vi "Process Build VI Operation.vi"(6 "Caller VI Path":path, 7 "Assert Scripting Configuration":T1, 8 "error in (no error)":errorcluster, 10 "Discard?":bool) -> (0 "error out":errorcluster, 3 "Assert VI Path":path, 5 "Valid Configuration":bool)   [LabVIEW 2016]
uses:
  Assert Scripting Configuration.ctl
  <vilib>/Utility/Data Type/Type Definitions/Data Type.ctl
  <vilib>/Utility/Data Type/NI_Data Type.lvlib
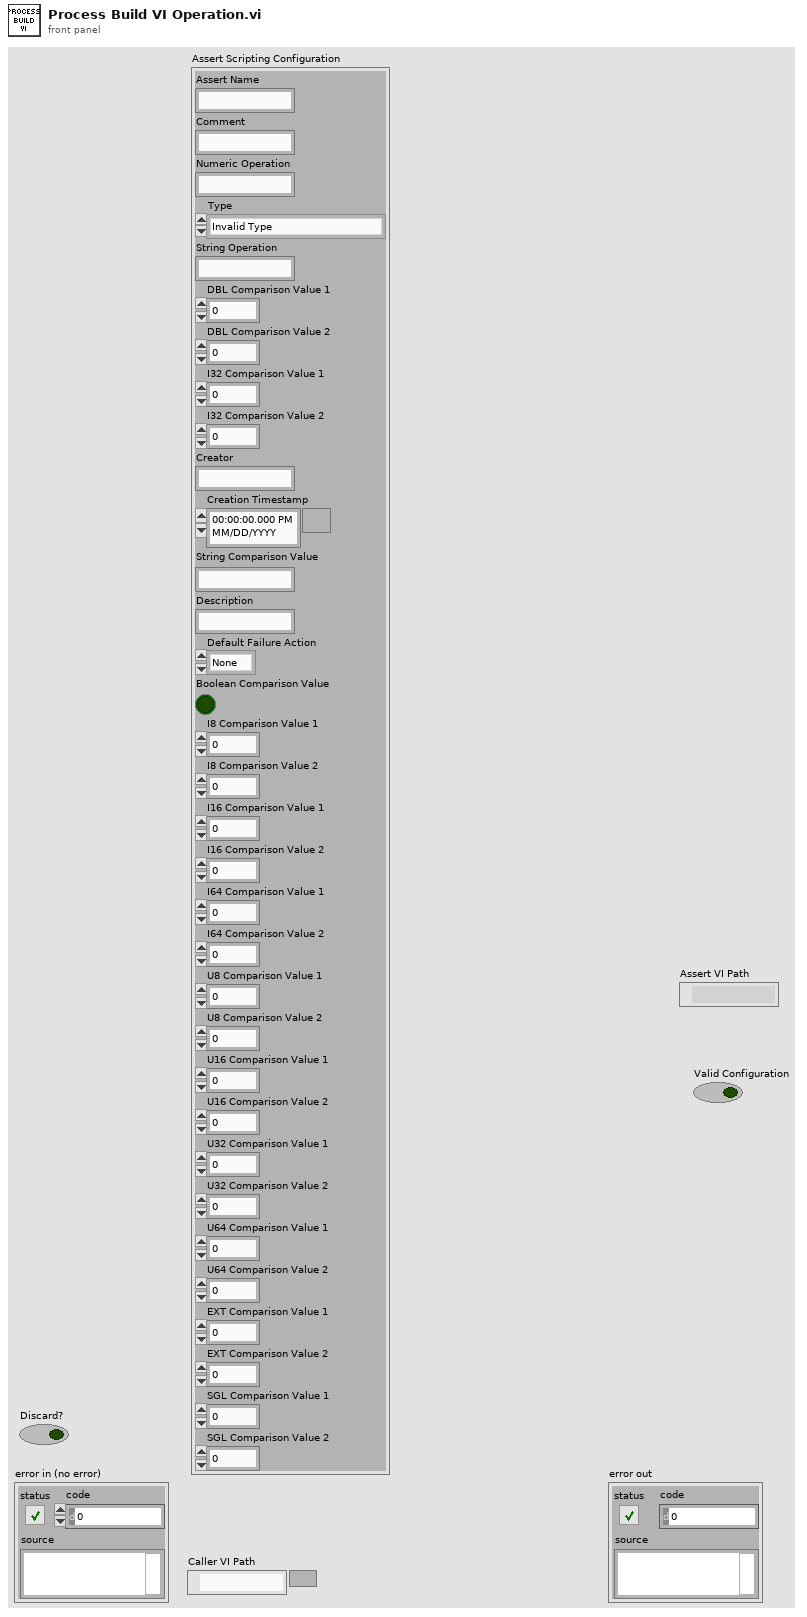
[diagram p1: front panel]
types:
  T1 = typedef "Assert Scripting Configuration.ctl" = cluster{"Assert Name":string, "Comment":string, "Numeric Operation":string, "Type":T2, "String Operation":string, "DBL Comparison Value 1":dbl, "DBL Comparison Value 2":dbl, "I32 Comparison Value 1":i32, "I32 Comparison Value 2":i32, "Creator":string, "Creation Timestamp":timestamp, "String Comparison Value":string, "Description":string, "Default Failure Action":enum16{"None", "Log To File", "Pause Execution", "Abort Execution"}, "Boolean Comparison Value":bool, "I8 Comparison Value 1":i8, "I8 Comparison Value 2":i8, "I16 Comparison Value 1":i16, "I16 Comparison Value 2":i16, "I64 Comparison Value 1":i64, "I64 Comparison Value 2":i64, "U8 Comparison Value 1":u8, "U8 Comparison Value 2":u8, "U16 Comparison Value 1":u16, "U16 Comparison Value 2":u16, "U32 Comparison Value 1":u32, "U32 Comparison Value 2":u32, "U64 Comparison Value 1":u64, "U64 Comparison Value 2":u64, "EXT Comparison Value 1":ext, "EXT Comparison Value 2":ext, "SGL Comparison Value 1":sgl, "SGL Comparison Value 2":sgl}
  T2 = typedef "NI_Data Type.lvlib/Data Type.ctl" = enum8{"Invalid Type", "Void", "I8", "I16", "I32", "I64", "U8", "U16", "U32", "U64", "Single Float", "Double Float", "Extended Float", "Single Complex", "Double Complex", "Extended Complex", "Enum U8", "Enum U16", "Enum U32", "Enum U64", "Single Float With Unit", "Double Float With Unit", "Extended Float With Unit", "Single Complex with Unit", "Double Complex with Unit", "Extended Complex with Unit", "Boolean", "String", "Path", "Picture", "Tag", "Array", "Cluster", "Variant", "LV Variant", "Waveform", "Timestamp", "Digital Waveform", "Digital Data", "ExpressData", "Refnum", "External Data", "VI", "Poly VI", "LabVIEW Class Instance", "Fixed Point"}
  T3 = enum16{"None", "Log To File", "Pause Execution", "Abort Execution"}
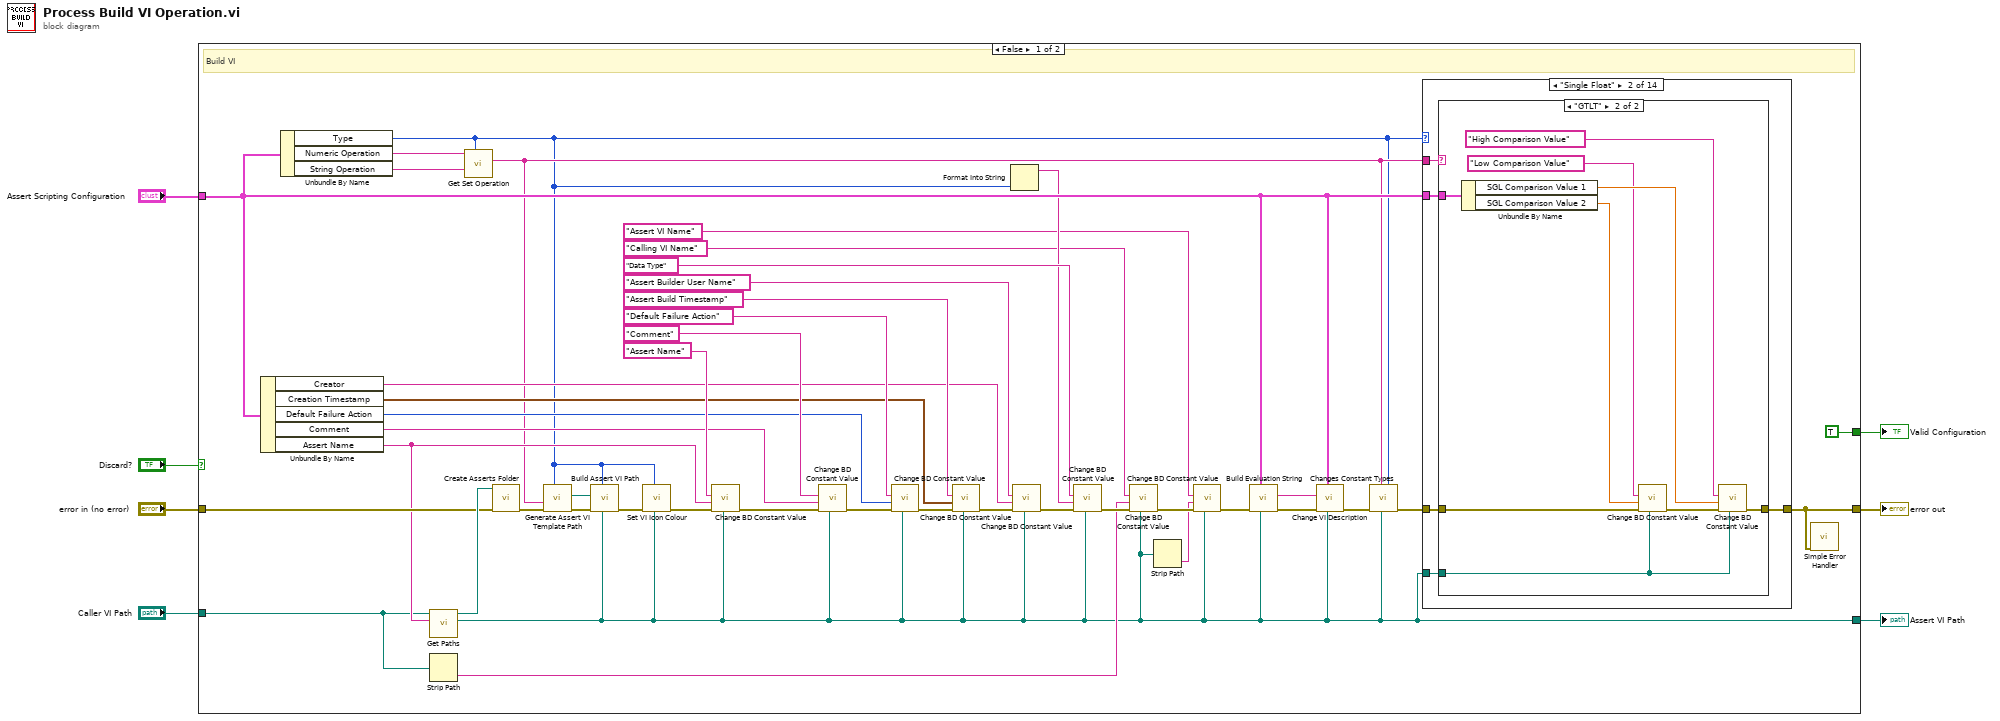
[diagram p0: block diagram]
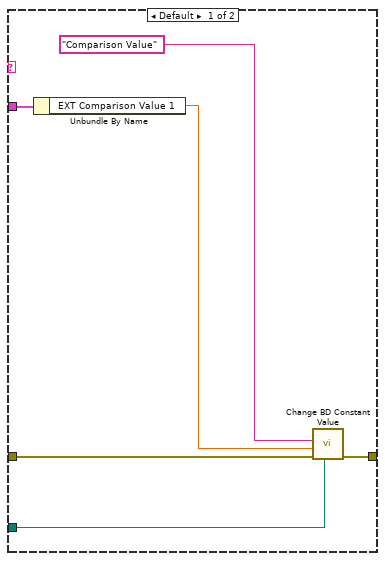
[diagram p3: hidden frame]
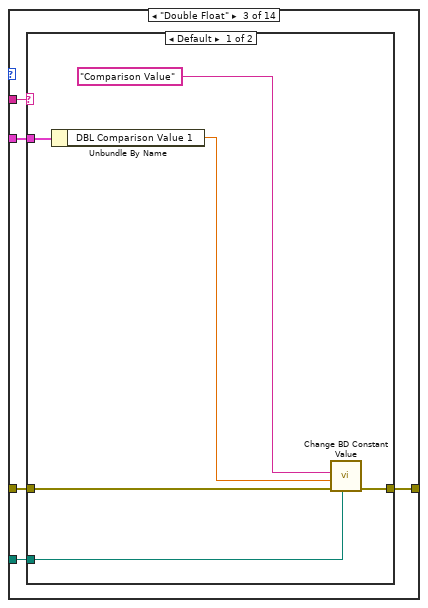
[diagram p4: hidden frame]
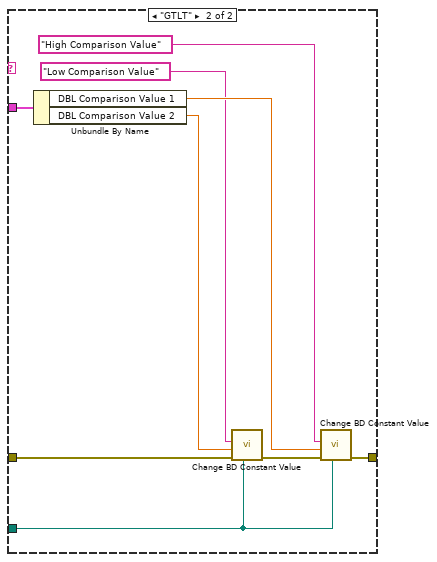
[diagram p5: hidden frame]
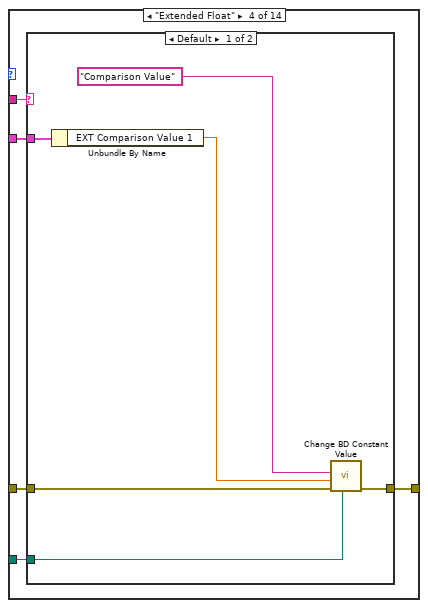
[diagram p6: hidden frame]
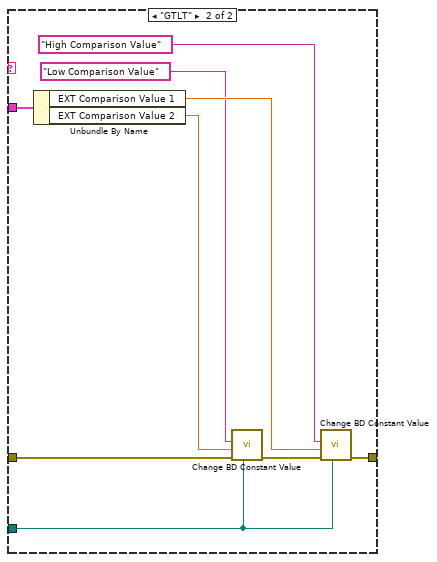
[diagram p7: hidden frame]
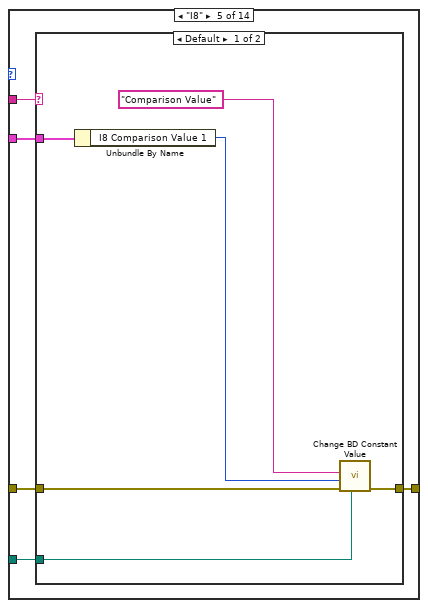
[diagram p8: hidden frame]
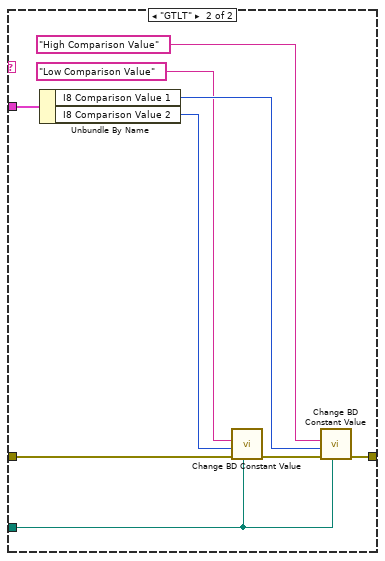
[diagram p9: hidden frame]
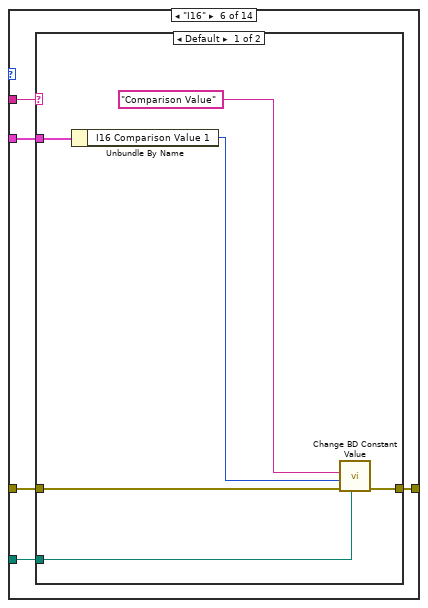
[diagram p10: hidden frame]
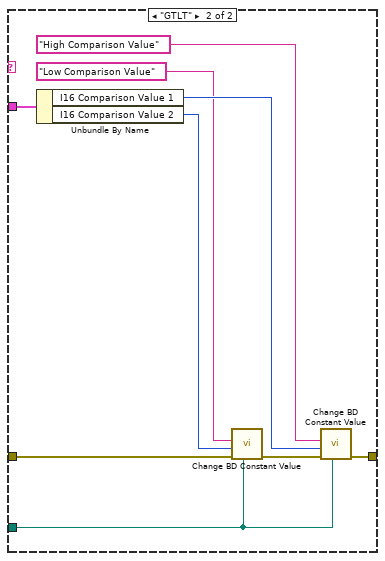
[diagram p11: hidden frame]
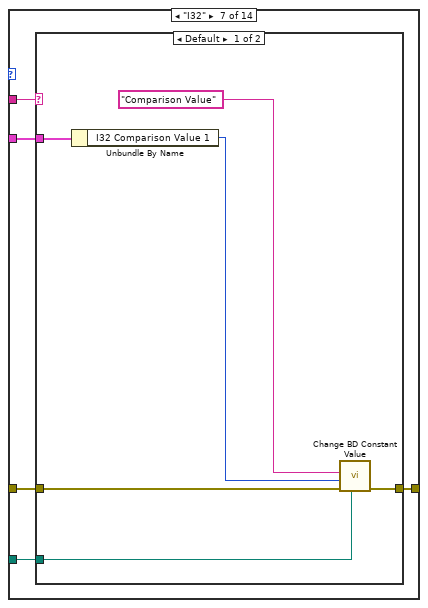
[diagram p12: hidden frame]
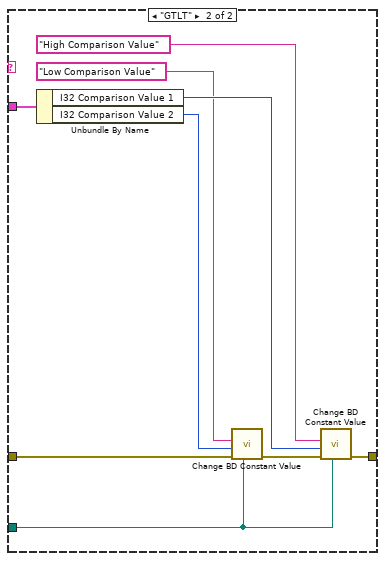
[diagram p13: hidden frame]
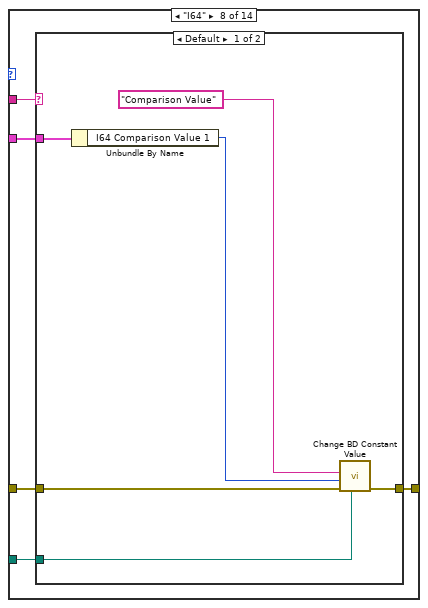
[diagram p14: hidden frame]
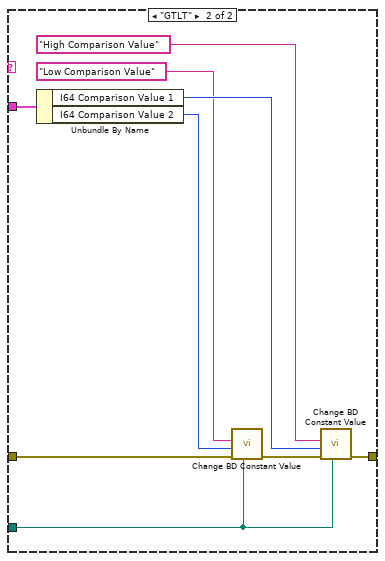
[diagram p15: hidden frame]
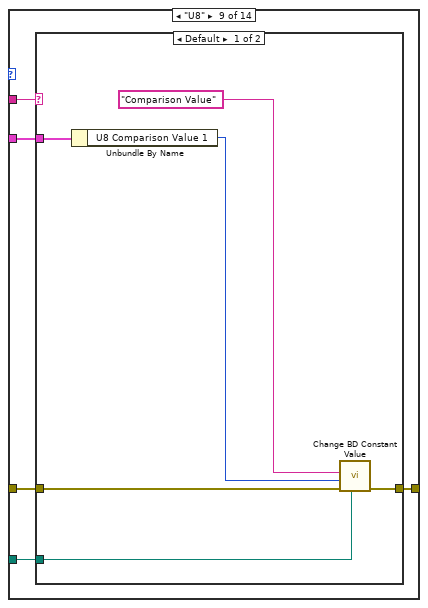
[diagram p16: hidden frame]
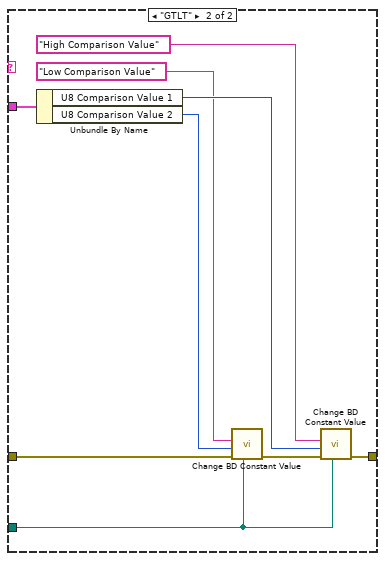
[diagram p17: hidden frame]
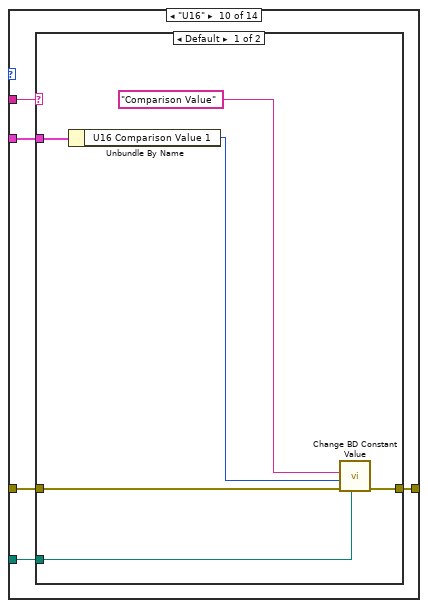
[diagram p18: hidden frame]
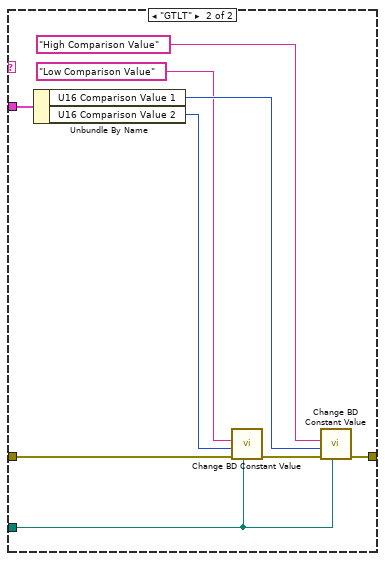
[diagram p19: hidden frame]
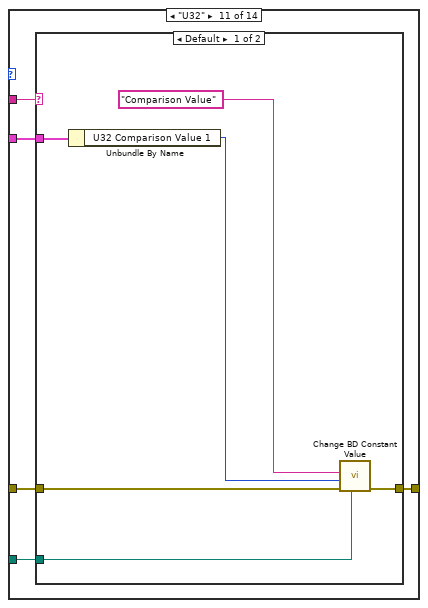
[diagram p20: hidden frame]
diagram:
  n1 = case shown="False" "Discard?" {
    tunnel: "error in (no error)" -> [w43 w285]
    tunnel: "Caller VI Path" -> [w15 _]
    tunnel: [w30 w285] -> w4
    tunnel: [w9 _] -> w5
    tunnel: [TRUE _] -> w6
    tunnel: "Assert Scripting Configuration" -> [w32 _]
    frame False {
      # "Build VI"
      n2 = Unbundle By Name(w32) -> ("Creator"=w21:string, "Creation Timestamp"=w22:timestamp, "Default Failure Action"=w34:T3, "Comment"=w37:string, "Assert Name"=w38:string)
      n3 = Unbundle By Name(w32) -> ("Type"=w8:T2, "Numeric Operation"=w40:string, "String Operation"=w39:string)
      n4 = call "Get Paths.vi"("Assert Name"=w38, "Path"=w15) -> ("Assert VI Path"=w9:path, "Asserts Folder Path"=w50:path)  [unwired: 8 in]
      n5 = Strip Path(path=w15) -> (name=w14:string)  [unwired: 1 out]
      n6 = call "Get Set Operation.vi"("Type"=w8, "String Operation"=w39, "Numeric Operation"=w40) -> ("Operation"=w10:string)  [unwired: 8 in]
      n7 = call "Create Asserts Folder.vi"("error in (no error)"=w43, "Folder Path"=w50) -> ("error out"=w44:errorcluster)  [unwired: 9 in]
      n8 = call "Generate Assert VI Template Path.vi"("Data Type"=w8, "error in (no error)"=w44, "Operation"=w10) -> ("error out"=w42:errorcluster, "Template Path"=w41:path)  [unwired: 7 in]
      n9 = call "Build Assert VI Path.vi"("Assert VI path"=w9, "Type"=w8, "error in (no error)"=w42, "Template Path"=w41) -> ("error out"=w51:errorcluster)  [unwired: 7 in]
      n10 = call "Set VI Icon Colour.vi"("VI Path"=w9, "Type"=w8, "error in (no error)"=w51) -> ("error out"=w13:errorcluster)  [unwired: 8 in]
      n11 = call "Change BD Constant Value.vi"("Assert VI Path"=w9, "error in (no error)"=w13, "Data Value"=w38, "Constant Name"="Assert Name") -> ("error out"=w46:errorcluster)  [unwired: 7 in]
      n12 = call "Change BD Constant Value.vi"("Assert VI Path"=w9, "error in (no error)"=w46, "Data Value"=w37, "Constant Name"="Comment") -> ("error out"=w45:errorcluster)  [unwired: 7 in]
      n13 = call "Change BD Constant Value.vi"("Assert VI Path"=w9, "error in (no error)"=w45, "Data Value"=w34, "Constant Name"="Default Failure Action") -> ("error out"=w36:errorcluster)  [unwired: 7 in]
      n14 = call "Change BD Constant Value.vi"("Assert VI Path"=w9, "error in (no error)"=w36, "Data Value"=w22, "Constant Name"="Assert Build Timestamp") -> ("error out"=w28:errorcluster)  [unwired: 7 in]
      n15 = Format Into String(w8) -> (resulting string=w23:string)  [unwired: 3 in, 1 out]
      n16 = call "Change BD Constant Value.vi"("Assert VI Path"=w9, "error in (no error)"=w28, "Data Value"=w21, "Constant Name"="Assert Builder User Name") -> ("error out"=w29:errorcluster)  [unwired: 7 in]
      n17 = call "Change BD Constant Value.vi"("Assert VI Path"=w9, "error in (no error)"=w29, "Data Value"=w23, "Constant Name"="Data Type") -> ("error out"=w27:errorcluster)  [unwired: 7 in]
      n18 = call "Change BD Constant Value.vi"("Assert VI Path"=w9, "error in (no error)"=w27, "Data Value"=w14, "Constant Name"="Calling VI Name") -> ("error out"=w20:errorcluster)  [unwired: 7 in]
      n19 = Strip Path(path=w9) -> (name=w16:string)  [unwired: 1 out]
      n20 = call "Change BD Constant Value.vi"("Assert VI Path"=w9, "error in (no error)"=w20, "Data Value"=w16, "Constant Name"="Assert VI Name") -> ("error out"=w19:errorcluster)  [unwired: 7 in]
      n21 = call "Build Evaluation String.vi"("VI Path"=w9, "Assert Scripting Configuration"=w32, "error in (no error)"=w19) -> ("error out"=w33:errorcluster, "Evaluation String"=w31:string)  [unwired: 7 in]
      n22 = call "Change VI Description.vi"("VI Path"=w9, "Assert Scripting Configuration"=w32, "error in (no error)"=w33, "Evaluation String"=w31) -> ("error out"=w12:errorcluster)  [unwired: 7 in]
      n23 = call "Changes Constant Types.vi"("Requested Data Type"=w8, "Assert VI Path"=w9, "String Control Name"=w10, "error in (no error)"=w12) -> ("error out"=w11:errorcluster)  [unwired: 7 in]
      n24 = case shown="\"Single Float\"" w8 {
        tunnel: w9 -> [_ w55 w75 w95 w117 w137 w157 w177 w197 w217 w237 w257 w274 w280]
        tunnel: w11 -> [w52 w56 w76 w96 w116 w136 w156 w176 w196 w216 w236 w256 w278 w284]
        tunnel: [w52 w57 w77 w97 w115 w135 w155 w175 w195 w215 w235 w255 w277 w283] -> w30
        tunnel: w32 -> [_ w54 w74 w94 w114 w134 w154 w174 w194 w214 w234 w254 w276 w282]
        tunnel: w10 -> [_ w53 w73 w93 w113 w133 w153 w173 w193 w213 w233 w253 _ _]
        frame Default {
        }
        frame "Single Float" {
          n25 = case shown="\"GTLT\"" w53 {
            tunnel: w55 -> [w58 w64]
            tunnel: w56 -> [w63 w72]
            tunnel: [w62 w68] -> w57
            tunnel: w54 -> [w61 w70]
            frame Default {
              n26 = Unbundle By Name(w61) -> ("EXT Comparison Value 1"=w60:ext)
              n27 = call "Change BD Constant Value.vi"("Assert VI Path"=w58, "error in (no error)"=w63, "Data Value"=w60, "Constant Name"="Comparison Value") -> ("error out"=w62:errorcluster)  [unwired: 7 in]
            }
            frame "GTLT" {
              n28 = Unbundle By Name(w70) -> ("SGL Comparison Value 1"=w67:sgl, "SGL Comparison Value 2"=w69:sgl)
              n29 = call "Change BD Constant Value.vi"("Assert VI Path"=w64, "error in (no error)"=w72, "Data Value"=w69, "Constant Name"="Low Comparison Value") -> ("error out"=w71:errorcluster)  [unwired: 7 in]
              n30 = call "Change BD Constant Value.vi"("Assert VI Path"=w64, "error in (no error)"=w71, "Data Value"=w67, "Constant Name"="High Comparison Value") -> ("error out"=w68:errorcluster)  [unwired: 7 in]
            }
          }
        }
        frame "Double Float" {
          n31 = case shown="Default" w73 {
            tunnel: w75 -> [w78 w84]
            tunnel: w76 -> [w83 w92]
            tunnel: [w82 w88] -> w77
            tunnel: w74 -> [w81 w90]
            frame Default {
              n32 = Unbundle By Name(w81) -> ("DBL Comparison Value 1"=w80:dbl)
              n33 = call "Change BD Constant Value.vi"("Assert VI Path"=w78, "error in (no error)"=w83, "Data Value"=w80, "Constant Name"="Comparison Value") -> ("error out"=w82:errorcluster)  [unwired: 7 in]
            }
            frame "GTLT" {
              n34 = Unbundle By Name(w90) -> ("DBL Comparison Value 1"=w87:dbl, "DBL Comparison Value 2"=w89:dbl)
              n35 = call "Change BD Constant Value.vi"("Assert VI Path"=w84, "error in (no error)"=w92, "Data Value"=w89, "Constant Name"="Low Comparison Value") -> ("error out"=w91:errorcluster)  [unwired: 7 in]
              n36 = call "Change BD Constant Value.vi"("Assert VI Path"=w84, "error in (no error)"=w91, "Data Value"=w87, "Constant Name"="High Comparison Value") -> ("error out"=w88:errorcluster)  [unwired: 7 in]
            }
          }
        }
        frame "Extended Float" {
          n37 = case shown="Default" w93 {
            tunnel: w95 -> [w98 w104]
            tunnel: w96 -> [w103 w112]
            tunnel: [w102 w108] -> w97
            tunnel: w94 -> [w101 w110]
            frame Default {
              n38 = Unbundle By Name(w101) -> ("EXT Comparison Value 1"=w100:ext)
              n39 = call "Change BD Constant Value.vi"("Assert VI Path"=w98, "error in (no error)"=w103, "Data Value"=w100, "Constant Name"="Comparison Value") -> ("error out"=w102:errorcluster)  [unwired: 7 in]
            }
            frame "GTLT" {
              n40 = Unbundle By Name(w110) -> ("EXT Comparison Value 1"=w107:ext, "EXT Comparison Value 2"=w109:ext)
              n41 = call "Change BD Constant Value.vi"("Assert VI Path"=w104, "error in (no error)"=w112, "Data Value"=w109, "Constant Name"="Low Comparison Value") -> ("error out"=w111:errorcluster)  [unwired: 7 in]
              n42 = call "Change BD Constant Value.vi"("Assert VI Path"=w104, "error in (no error)"=w111, "Data Value"=w107, "Constant Name"="High Comparison Value") -> ("error out"=w108:errorcluster)  [unwired: 7 in]
            }
          }
        }
        frame "I8" {
          n43 = case shown="Default" w113 {
            tunnel: w117 -> [w118 w124]
            tunnel: w116 -> [w123 w132]
            tunnel: [w122 w128] -> w115
            tunnel: w114 -> [w121 w130]
            frame Default {
              n44 = Unbundle By Name(w121) -> ("I8 Comparison Value 1"=w120:i8)
              n45 = call "Change BD Constant Value.vi"("Assert VI Path"=w118, "error in (no error)"=w123, "Data Value"=w120, "Constant Name"="Comparison Value") -> ("error out"=w122:errorcluster)  [unwired: 7 in]
            }
            frame "GTLT" {
              n46 = Unbundle By Name(w130) -> ("I8 Comparison Value 1"=w127:i8, "I8 Comparison Value 2"=w129:i8)
              n47 = call "Change BD Constant Value.vi"("Assert VI Path"=w124, "error in (no error)"=w132, "Data Value"=w129, "Constant Name"="Low Comparison Value") -> ("error out"=w131:errorcluster)  [unwired: 7 in]
              n48 = call "Change BD Constant Value.vi"("Assert VI Path"=w124, "error in (no error)"=w131, "Data Value"=w127, "Constant Name"="High Comparison Value") -> ("error out"=w128:errorcluster)  [unwired: 7 in]
            }
          }
        }
        frame "I16" {
          n49 = case shown="Default" w133 {
            tunnel: w137 -> [w138 w144]
            tunnel: w136 -> [w143 w152]
            tunnel: [w142 w148] -> w135
            tunnel: w134 -> [w141 w150]
            frame Default {
              n50 = Unbundle By Name(w141) -> ("I16 Comparison Value 1"=w140:i16)
              n51 = call "Change BD Constant Value.vi"("Assert VI Path"=w138, "error in (no error)"=w143, "Data Value"=w140, "Constant Name"="Comparison Value") -> ("error out"=w142:errorcluster)  [unwired: 7 in]
            }
            frame "GTLT" {
              n52 = Unbundle By Name(w150) -> ("I16 Comparison Value 1"=w147:i16, "I16 Comparison Value 2"=w149:i16)
              n53 = call "Change BD Constant Value.vi"("Assert VI Path"=w144, "error in (no error)"=w152, "Data Value"=w149, "Constant Name"="Low Comparison Value") -> ("error out"=w151:errorcluster)  [unwired: 7 in]
              n54 = call "Change BD Constant Value.vi"("Assert VI Path"=w144, "error in (no error)"=w151, "Data Value"=w147, "Constant Name"="High Comparison Value") -> ("error out"=w148:errorcluster)  [unwired: 7 in]
            }
          }
        }
        frame "I32" {
          n55 = case shown="Default" w153 {
            tunnel: w157 -> [w158 w164]
            tunnel: w156 -> [w163 w172]
            tunnel: [w162 w168] -> w155
            tunnel: w154 -> [w161 w170]
            frame Default {
              n56 = Unbundle By Name(w161) -> ("I32 Comparison Value 1"=w160:i32)
              n57 = call "Change BD Constant Value.vi"("Assert VI Path"=w158, "error in (no error)"=w163, "Data Value"=w160, "Constant Name"="Comparison Value") -> ("error out"=w162:errorcluster)  [unwired: 7 in]
            }
            frame "GTLT" {
              n58 = Unbundle By Name(w170) -> ("I32 Comparison Value 1"=w167:i32, "I32 Comparison Value 2"=w169:i32)
              n59 = call "Change BD Constant Value.vi"("Assert VI Path"=w164, "error in (no error)"=w172, "Data Value"=w169, "Constant Name"="Low Comparison Value") -> ("error out"=w171:errorcluster)  [unwired: 7 in]
              n60 = call "Change BD Constant Value.vi"("Assert VI Path"=w164, "error in (no error)"=w171, "Data Value"=w167, "Constant Name"="High Comparison Value") -> ("error out"=w168:errorcluster)  [unwired: 7 in]
            }
          }
        }
        frame "I64" {
          n61 = case shown="Default" w173 {
            tunnel: w177 -> [w178 w184]
            tunnel: w176 -> [w183 w192]
            tunnel: [w182 w188] -> w175
            tunnel: w174 -> [w181 w190]
            frame Default {
              n62 = Unbundle By Name(w181) -> ("I64 Comparison Value 1"=w180:i64)
              n63 = call "Change BD Constant Value.vi"("Assert VI Path"=w178, "error in (no error)"=w183, "Data Value"=w180, "Constant Name"="Comparison Value") -> ("error out"=w182:errorcluster)  [unwired: 7 in]
            }
            frame "GTLT" {
              n64 = Unbundle By Name(w190) -> ("I64 Comparison Value 1"=w187:i64, "I64 Comparison Value 2"=w189:i64)
              n65 = call "Change BD Constant Value.vi"("Assert VI Path"=w184, "error in (no error)"=w192, "Data Value"=w189, "Constant Name"="Low Comparison Value") -> ("error out"=w191:errorcluster)  [unwired: 7 in]
              n66 = call "Change BD Constant Value.vi"("Assert VI Path"=w184, "error in (no error)"=w191, "Data Value"=w187, "Constant Name"="High Comparison Value") -> ("error out"=w188:errorcluster)  [unwired: 7 in]
            }
          }
        }
        frame "U8" {
          n67 = case shown="Default" w193 {
            tunnel: w197 -> [w198 w204]
            tunnel: w196 -> [w203 w212]
            tunnel: [w202 w208] -> w195
            tunnel: w194 -> [w201 w210]
            frame Default {
              n68 = Unbundle By Name(w201) -> ("U8 Comparison Value 1"=w200:u8)
              n69 = call "Change BD Constant Value.vi"("Assert VI Path"=w198, "error in (no error)"=w203, "Data Value"=w200, "Constant Name"="Comparison Value") -> ("error out"=w202:errorcluster)  [unwired: 7 in]
            }
            frame "GTLT" {
              n70 = Unbundle By Name(w210) -> ("U8 Comparison Value 1"=w207:u8, "U8 Comparison Value 2"=w209:u8)
              n71 = call "Change BD Constant Value.vi"("Assert VI Path"=w204, "error in (no error)"=w212, "Data Value"=w209, "Constant Name"="Low Comparison Value") -> ("error out"=w211:errorcluster)  [unwired: 7 in]
              n72 = call "Change BD Constant Value.vi"("Assert VI Path"=w204, "error in (no error)"=w211, "Data Value"=w207, "Constant Name"="High Comparison Value") -> ("error out"=w208:errorcluster)  [unwired: 7 in]
            }
          }
        }
        frame "U16" {
          n73 = case shown="Default" w213 {
            tunnel: w217 -> [w218 w224]
            tunnel: w216 -> [w223 w232]
            tunnel: [w222 w228] -> w215
            tunnel: w214 -> [w221 w230]
            frame Default {
              n74 = Unbundle By Name(w221) -> ("U16 Comparison Value 1"=w220:u16)
              n75 = call "Change BD Constant Value.vi"("Assert VI Path"=w218, "error in (no error)"=w223, "Data Value"=w220, "Constant Name"="Comparison Value") -> ("error out"=w222:errorcluster)  [unwired: 7 in]
            }
            frame "GTLT" {
              n76 = Unbundle By Name(w230) -> ("U16 Comparison Value 1"=w227:u16, "U16 Comparison Value 2"=w229:u16)
              n77 = call "Change BD Constant Value.vi"("Assert VI Path"=w224, "error in (no error)"=w232, "Data Value"=w229, "Constant Name"="Low Comparison Value") -> ("error out"=w231:errorcluster)  [unwired: 7 in]
              n78 = call "Change BD Constant Value.vi"("Assert VI Path"=w224, "error in (no error)"=w231, "Data Value"=w227, "Constant Name"="High Comparison Value") -> ("error out"=w228:errorcluster)  [unwired: 7 in]
            }
          }
        }
        frame "U32" {
          n79 = case shown="Default" w233 {
            tunnel: w237 -> [w238 w244]
            tunnel: w236 -> [w243 w252]
            tunnel: [w242 w248] -> w235
            tunnel: w234 -> [w241 w250]
            frame Default {
              n80 = Unbundle By Name(w241) -> ("U32 Comparison Value 1"=w240:u32)
              n81 = call "Change BD Constant Value.vi"("Assert VI Path"=w238, "error in (no error)"=w243, "Data Value"=w240, "Constant Name"="Comparison Value") -> ("error out"=w242:errorcluster)  [unwired: 7 in]
            }
            frame "GTLT" {
              n82 = Unbundle By Name(w250) -> ("U32 Comparison Value 1"=w247:u32, "U32 Comparison Value 2"=w249:u32)
              n83 = call "Change BD Constant Value.vi"("Assert VI Path"=w244, "error in (no error)"=w252, "Data Value"=w249, "Constant Name"="Low Comparison Value") -> ("error out"=w251:errorcluster)  [unwired: 7 in]
              n84 = call "Change BD Constant Value.vi"("Assert VI Path"=w244, "error in (no error)"=w251, "Data Value"=w247, "Constant Name"="High Comparison Value") -> ("error out"=w248:errorcluster)  [unwired: 7 in]
            }
          }
        }
        frame "U64" {
          n85 = case shown="Default" w253 {
            tunnel: w257 -> [w258 w264]
            tunnel: w256 -> [w263 w272]
            tunnel: [w262 w268] -> w255
            tunnel: w254 -> [w261 w270]
            frame Default {
              n86 = Unbundle By Name(w261) -> ("U64 Comparison Value 1"=w260:u64)
              n87 = call "Change BD Constant Value.vi"("Assert VI Path"=w258, "error in (no error)"=w263, "Data Value"=w260, "Constant Name"="Comparison Value") -> ("error out"=w262:errorcluster)  [unwired: 7 in]
            }
            frame "GTLT" {
              n88 = Unbundle By Name(w270) -> ("U64 Comparison Value 1"=w267:u64, "U64 Comparison Value 2"=w269:u64)
              n89 = call "Change BD Constant Value.vi"("Assert VI Path"=w264, "error in (no error)"=w272, "Data Value"=w269, "Constant Name"="Low Comparison Value") -> ("error out"=w271:errorcluster)  [unwired: 7 in]
              n90 = call "Change BD Constant Value.vi"("Assert VI Path"=w264, "error in (no error)"=w271, "Data Value"=w267, "Constant Name"="High Comparison Value") -> ("error out"=w268:errorcluster)  [unwired: 7 in]
            }
          }
        }
        frame "String" {
          n91 = Unbundle By Name(w276) -> ("String Comparison Value"=w275:string)
          n92 = call "Change BD Constant Value.vi"("Assert VI Path"=w274, "error in (no error)"=w278, "Data Value"=w275, "Constant Name"="Comparison Value") -> ("error out"=w277:errorcluster)  [unwired: 7 in]
        }
        frame "Boolean" {
          n93 = Unbundle By Name(w282) -> ("Boolean Comparison Value"=w281:bool)
          n94 = call "Change BD Constant Value.vi"("Assert VI Path"=w280, "error in (no error)"=w284, "Data Value"=w281, "Constant Name"="Comparison Value") -> ("error out"=w283:errorcluster)  [unwired: 7 in]
        }
      }
      n95 = call <vilib>:"Simple Error Handler.vi"("error in (no error)"=w30) -> ()  [unwired: 4 in, 5 out]
    }
    frame True {
      # "Cancelled"
    }
  }
  "Valid Configuration" <- w6
  "Assert VI Path" <- w5
  "error out" <- w4
